vi "init_hw.vi"(8 "error in (no error)":errorcluster, 11 "_camera in":refnum<class "_camera.lvclass">) -> (0 "error out":errorcluster, 2 "success ?":bool=TRUE, 3 "_camera out":refnum<class "_camera.lvclass">)   [LabVIEW 2019, in "_camera.lvlib" / "_camera.lvclass"]
uses:
  _camera.lvclass
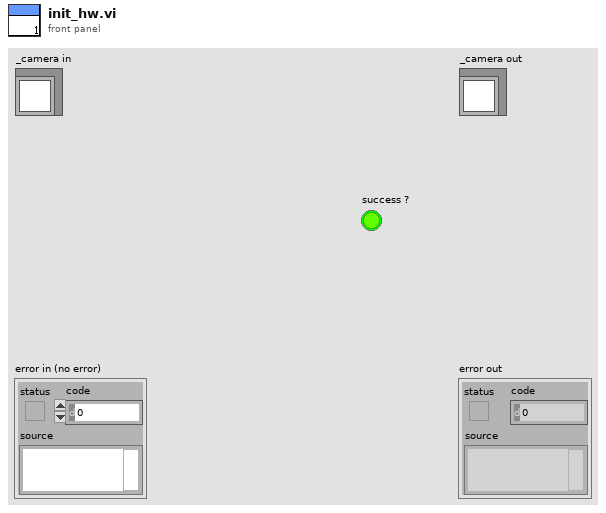
[diagram p1: front panel]
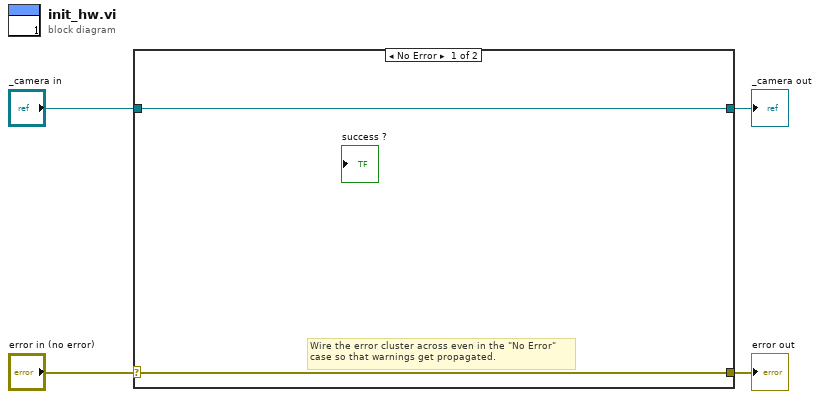
[diagram p0: block diagram]
diagram:
  n1 = case shown="No Error" "error in (no error)" {
    selector: "error in (no error)" -> [w5 w8]
    tunnel: [w5 w8] -> w3
    tunnel: [w6 w7] -> w1
    tunnel: "_camera in" -> [w6 w7]
    frame No Error {
      # "Wire the error cluster across even in the \"No Error\"\ncase so that warnings get propagated."
    }
    frame Error {
    }
  }
  "error out" <- w3
  "_camera out" <- w1
